vi "PosStrikerAnguloGol.vi"(9 "atacando contra":bool, 10 "IA State":T1={"our_robots"=[], "enemy_robots"=[], "balls"=[], "geometry"={"line_width"=0, "field_length"=0, "field_width"=0, "boundary_width"=0, "referee_width"=0, "goal_width"=0, "goal_depth"=0, "goal_wall_width"=0, "center_circle_radius"=0, "defense_radius"=0, "defense_stretch"=0, "free_kick_from_defense_dist"=0, "penalty_spot_from_field_line_dist"=0, "penalty_line_from_spot_dist"=0}, "IA Judge"={"stage"="", "command"="", "our_goalie_id"=0.0, "enemy_goalie_id"=0.0, "command enum"=enum."Halt", "Time"=enum."Azul"}, "Received Timestamp"=timestamp(0 s since 1904-01-01), "Events"={"Touch"=FALSE, "Ball out"=FALSE, "id touch"=0.0, "Ball out of \nVision"=FALSE, "Ball inside \nGoalie area"=FALSE, "Robot not responding"=FALSE, "Robots responding status"=[1.0, 1.0, 1.0, 1.0, 1.0, 1.0], "Enemy Ball \nPossession"=FALSE, "Pass State"=FALSE, "id end of pass"=0.0, "Kick"=FALSE, "Id ini Possession"=0.0, "Ball Possesion"=FALSE, "Id Possesion"=0.0}}) -> (2 "theta final":dbl)   [LabVIEW 2017]
uses:
  Core/AI Input.ctl
  Core/AI Robot.ctl
  Intel/Functions Enum.ctl
  Intel/AttackerStates.ctl
  Core/AI Ball.ctl
  Core/Field Size.ctl
  Core/AI Judge.ctl
  Intel/Command Enum.ctl
  Events/Events.ctl
panel:
  in  "XdoAttacker":dbl
  in  "YdoAttacker":dbl
  in  "Array":dbl[](array[numeric])=[0.0, 0.0, 0.0, 0.0, 0.0, 0.0]
  in  "Contador 2":dbl
  in  "fim do intervalo":dbl=-1.57
  in  "inicio do intervalo":dbl=-1.57
  in  "tamanho do intervalo":dbl
  in  "valor de theta":dbl
  in  "RobôsParaAnalisar":dbl[][](array[numeric])=[[99999.0, 99999.0], [99999.0, 99999.0], [99999.0, 99999.0], [99999.0, 99999.0], [99999.0, 99999.0], [99999.0, 99999.0], [99999.0, 99999.0]]
  in  "Contador":dbl
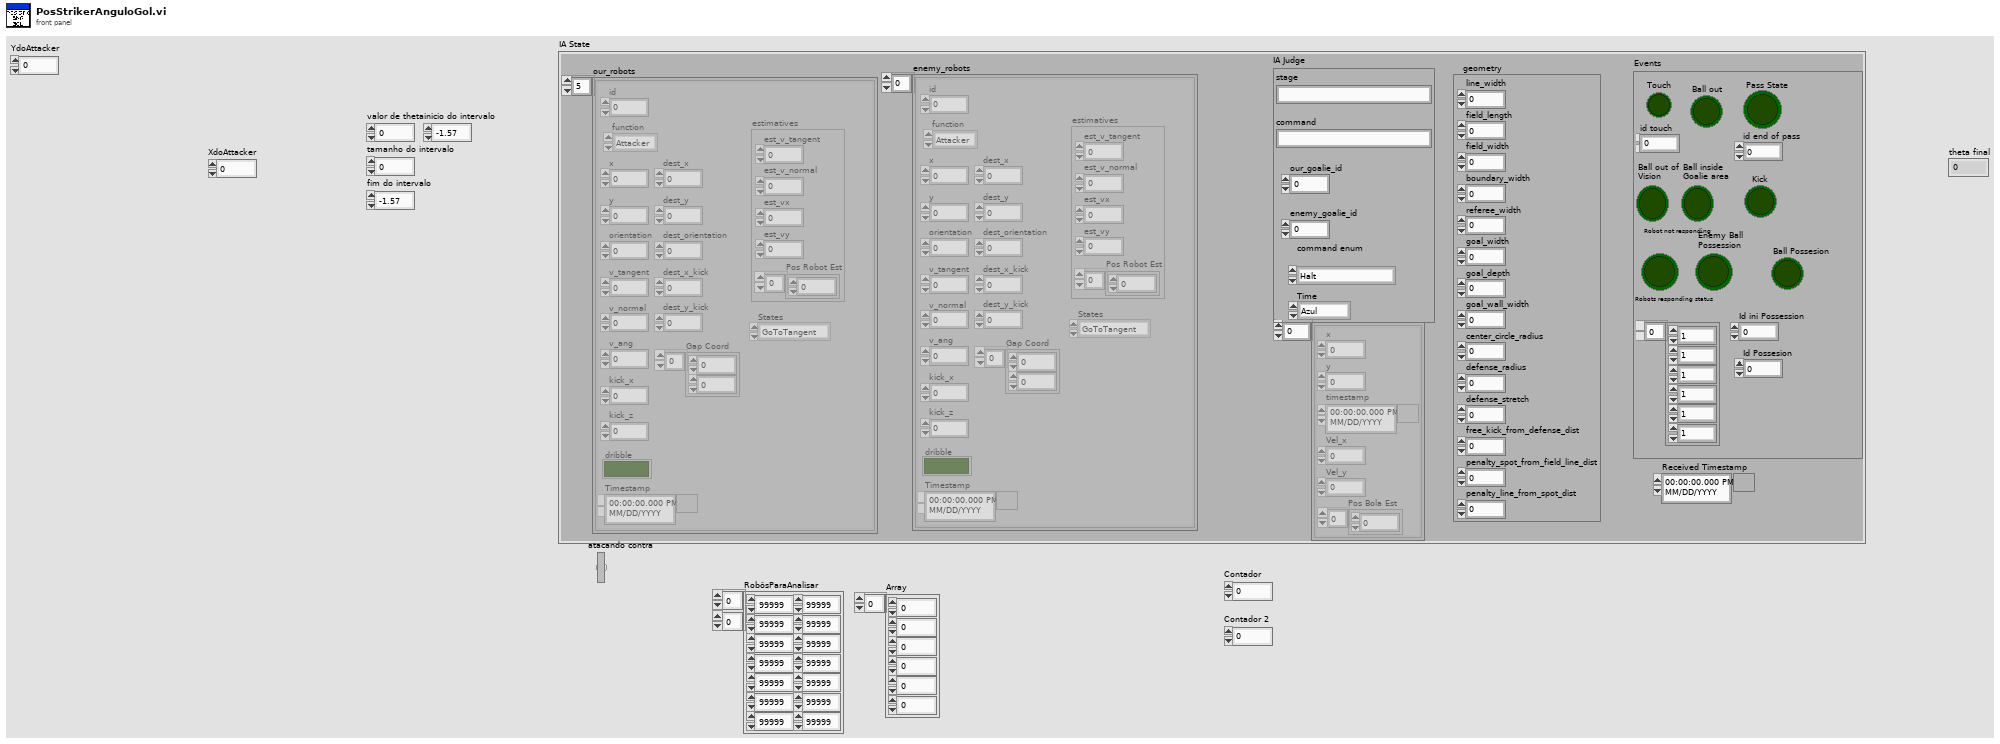
[diagram p1: front panel]
types:
  T1 = typedef "AI Input.ctl" = cluster{"our_robots":T2[], "enemy_robots":T2[], "balls":T5[], "geometry":T6, "IA Judge":T7, "Received Timestamp":timestamp, "Events":T9}
  T2 = typedef "AI Robot.ctl" = cluster{"id":u32, "function":T3, "x":dbl, "y":dbl, "orientation":dbl, "v_tangent":dbl, "v_normal":dbl, "v_ang":dbl, "kick_x":dbl, "kick_z":dbl, "dribble":bool, "Timestamp":timestamp, "dest_x":dbl, "dest_y":dbl, "dest_orientation":dbl, "estimatives":cluster{"est_v_tangent":dbl, "est_v_normal":dbl, "est_vx":dbl, "est_vy":dbl, "Pos Robot Est":dbl[]}, "dest_x_kick":dbl, "dest_y_kick":dbl, "Gap Coord":dbl[], "States":T4}
  T3 = typedef "Functions Enum.ctl" = enum16{"Attacker", "Goalie", "Defender", "Striker", "Goto 0", "Dummy", "Kicker", "ZigZag"}
  T4 = typedef "AttackerStates.ctl" = enum16{"Pass", "GoToTangent", "BallGetting", "GoToKick", ""}
  T5 = typedef "AI Ball.ctl" = cluster{"x":dbl, "y":dbl, "timestamp":timestamp, "Vel_x":dbl, "Vel_y":dbl, "Pos Bola Est":dbl[]}
  T6 = typedef "Field Size.ctl" = cluster{"line_width":u32, "field_length":u32, "field_width":u32, "boundary_width":u32, "referee_width":u32, "goal_width":u32, "goal_depth":u32, "goal_wall_width":u32, "center_circle_radius":u32, "defense_radius":u32, "defense_stretch":u32, "free_kick_from_defense_dist":u32, "penalty_spot_from_field_line_dist":u32, "penalty_line_from_spot_dist":u32}
  T7 = typedef "AI Judge.ctl" = cluster{"stage":string, "command":string, "our_goalie_id":dbl, "enemy_goalie_id":dbl, "command enum":T8, "Time":enum16{"Azul", "Amarelo"}}
  T8 = typedef "Command Enum.ctl" = enum16{"Halt", "Stop", "Force Start", "PKA Normal Start", "Prepare Kickoff Ally", "PKE Normal Start", "Prepare Kickoff Enemy", "Prepare Penalty Ally", "PPA Normal Start", "Prepare Penalty Enemy", "PPE Normal Start", "Direct Free Enemy", "Direct Free Ally", "Indirect Free Enemy", "Indirect Free Ally", "Timeout Enemy", "Timeout Ally", "Goal Enemy", "Goal Ally", "Ball Placement Enemy", "Ball Placement Ally", "Normal Half Time", "Extra Time Break", "Extra Half Time", "None", "Post Game"}
  T9 = typedef "Events.ctl" = cluster{"Touch":bool, "Ball out":bool, "id touch":dbl, "Ball out of \nVision":bool, "Ball inside \nGoalie area":bool, "Robot not responding":bool, "Robots responding status":dbl[], "Enemy Ball \nPossession":bool, "Pass State":bool, "id end of pass":dbl, "Kick":bool, "Id ini Possession":dbl, "Ball Possesion":bool, "Id Possesion":dbl}
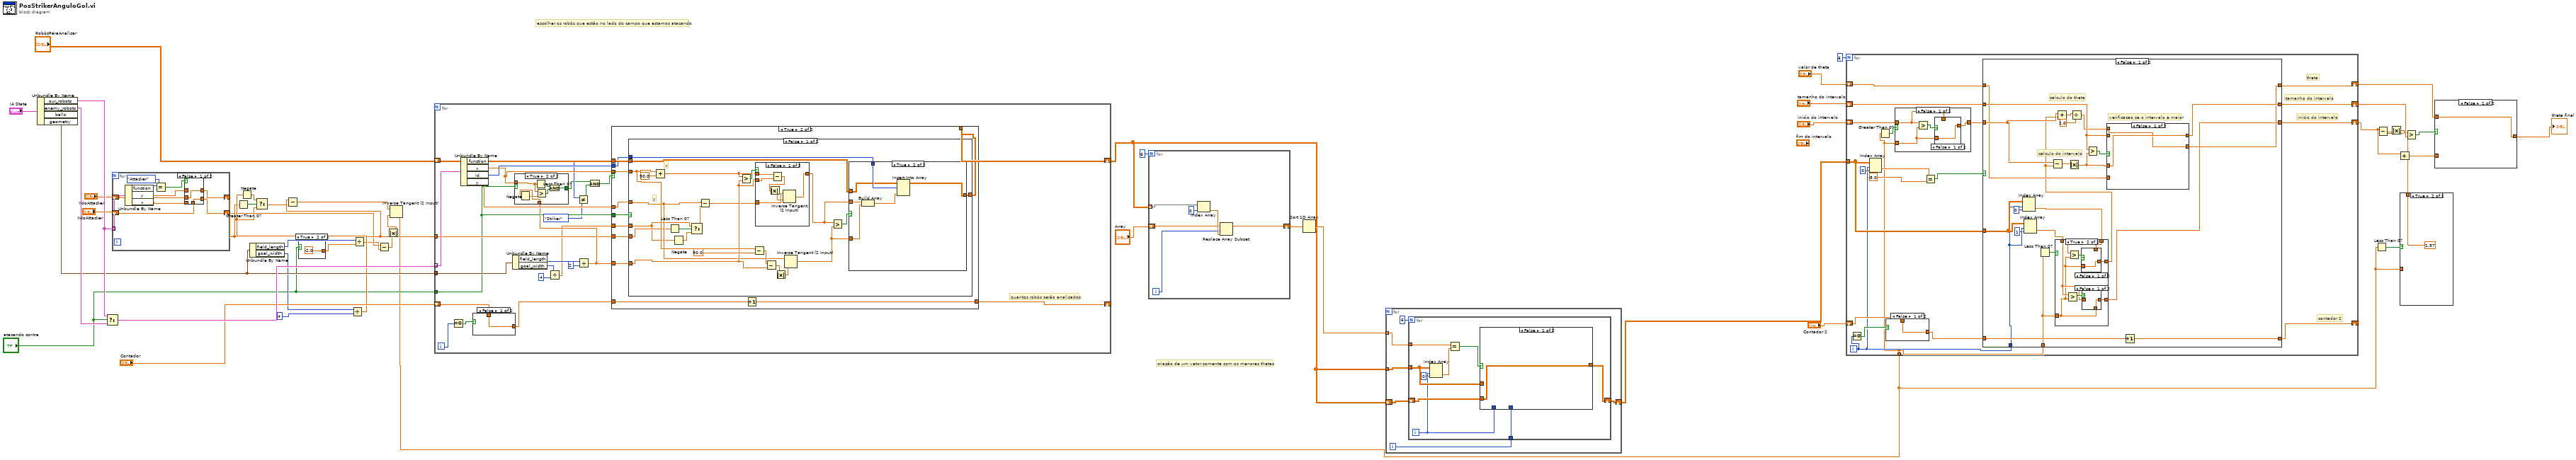
[diagram p0: block diagram]
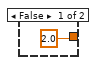
[diagram p3: hidden frame]
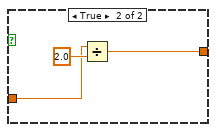
[diagram p5: hidden frame]
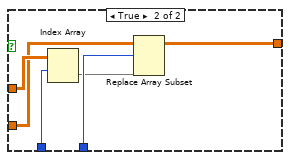
[diagram p6: hidden frame]
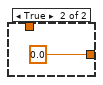
[diagram p9: hidden frame]
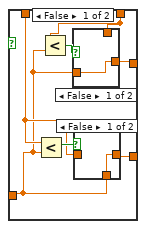
[diagram p10: hidden frame]
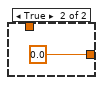
[diagram p17: hidden frame]
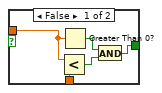
[diagram p18: hidden frame]
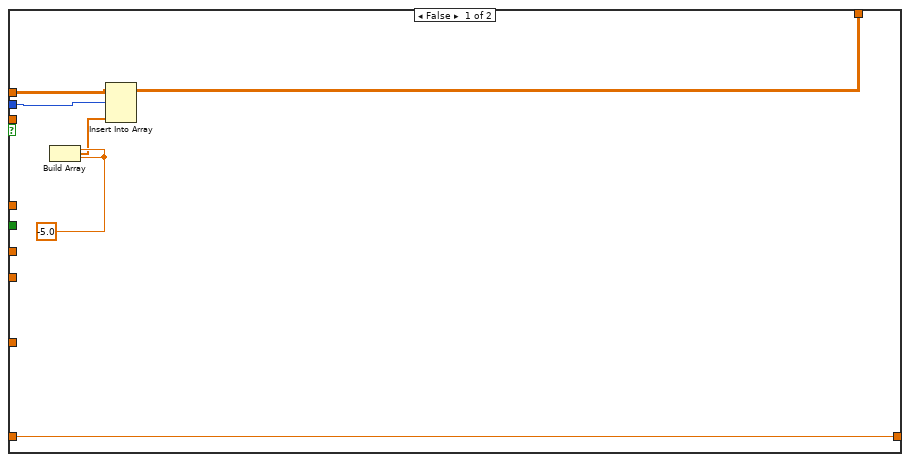
[diagram p19: hidden frame]
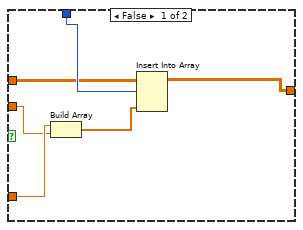
[diagram p20: hidden frame]
diagram:
  # "criação de um vetor somente com os menores thetas"
  # "escolher os robôs que estão no lado do campo que estamos atacando"
  n1 = Unbundle By Name("IA State") -> ("our_robots"=w21:T2[], "enemy_robots"=w45:T2[], "geometry"=w18:T6)  [unwired: 1 out]
  n2 = Select(t=w21, s="atacando contra", f=w45) -> (s? t:f=w44:T2[])
  n3 = for {
    tunnel: w21 -> [w56] mode=indexing
    shift-right: [w51] -> w11
    shift-left: "YdoAttacker" -> [w50]
    shift-right: [w48] -> w8
    shift-left: "XdoAttacker" -> [w47]
    n4 = Unbundle By Name(w56) -> ("function"=w55:T3, "y"=w52:dbl, "x"=w49:dbl)
    n5 = Equal?(x=w55, y=Functions_Enum."Attacker") -> (x = y?=w53:bool)
    n6 = case shown="False" w53 {
      tunnel: w52 -> [_ w60]
      tunnel: [w58 w60] -> w51
      tunnel: w50 -> [w58 _]
      tunnel: w49 -> [_ w59]
      tunnel: [w57 w59] -> w48
      tunnel: w47 -> [w57 _]
      frame False {
      }
      frame True {
      }
    }
  }
  n7 = Greater Than 0?(x=w11) -> (x > 0?=w14:bool)
  n8 = Unbundle By Name(w18) -> ("field_length"=w15:u32, "goal_width"=w17:u32)
  n9 = case shown="True" "atacando contra" {
    tunnel: [2.0 ("y") -2.0 ("y")] -> w6
    frame False {
    }
    frame True {
    }
  }
  n10 = Divide(x=w17, y=u32 4) -> (x/y=w12:dbl)
  n11 = Negate(x=w12) -> (-x=w13:dbl)
  n12 = Select(t=w13, s=w14, f=w12) -> (s? t:f=w10:dbl)
  n13 = Subtract(x=w11, y=w10) -> (x-y=w7:dbl)
  n14 = Divide(x=w15, y=w6) -> (x/y=w9:dbl)
  n15 = Subtract(x=w8, y=w9) -> (x-y=w2:dbl)
  n16 = Absolute Value(x=w2) -> (abs(x)=w1:dbl)
  n17 = Inverse Tangent (2 Input)(1:w1, 2:w7) -> (0:w3:dbl)
  n18 = for {
    tunnel: w44 -> [w87] mode=indexing
    tunnel: "atacando contra" -> [w69]
    shift-right: [w77] -> w32
    shift-left: "RobôsParaAnalisar" -> [w86]
    shift-right: [w78] -> _
    shift-left: "Contador" -> [w80]
    tunnel: w18 -> [w70]
    tunnel: w11 -> [w74]
    i -> [w81]
    # "quantos robôs serão analisados"
    n19 = Equal To 0?(x=w81) -> (x = 0?=w82:bool)
    n20 = Unbundle By Name(w87) -> ("function"=w67:T3, "x"=w84:dbl, "id"=w85:u32, "y"=w83:dbl)
    n21 = case shown="False" w82 {
      tunnel: w80 -> [w88 _]
      tunnel: [w88 0.0] -> w79
      frame False {
      }
      frame True {
      }
    }
    n22 = Unbundle By Name(w70) -> ("field_length"=w76:u32, "goal_width"=w73:u32)
    n23 = Divide(x=w73, y=u32 4) -> (x/y=w71:dbl)
    n24 = Not Equal?(x=w67, y=Functions_Enum."Striker") -> (x != y?=w64:bool)
    n25 = Divide(x=w76, y=u32 2) -> (x/y=w75:dbl)
    n26 = case shown="True" w69 {
      tunnel: w84 -> [w94 w95]
      tunnel: [w90 w100] -> w63
      tunnel: w75 -> [w93 w96]
      frame False {
        n27 = Less?(x=w94, y=w93) -> (x < y?=w91:bool)
        n28 = Greater Than 0?(x=w94) -> (x > 0?=w92:bool)
        n29 = And(x=w92, y=w91) -> (x .and. y?=w90:bool)
      }
      frame True {
        n30 = Negate(x=w96) -> (-x=w97:dbl)
        n31 = Less Than 0?(x=w95) -> (x < 0?=w99:bool)
        n32 = Greater?(x=w95, y=w97) -> (0:w98:bool)
        n33 = And(x=w99, y=w98) -> (x .and. y?=w100:bool)
      }
    }
    n34 = And(x=w63, y=w64) -> (x .and. y?=w65:bool)
    n35 = case shown="True" w65 {
      tunnel: w86 -> [w105 w112]
      tunnel: w85 -> [w104 w110]
      tunnel: w84 -> [_ w114]
      tunnel: w83 -> [_ w111]
      tunnel: w79 -> [w106 w116]
      tunnel: [w106 w117] -> w78
      tunnel: [w101 w109] -> w77
      tunnel: w69 -> [_ w115]
      tunnel: w75 -> [_ w113]
      tunnel: w74 -> [_ w108]
      tunnel: w71 -> [_ w107]
      frame False {
        w103 = -5.0 ("element")
        n36 = Build Array(w103, w103) -> (w102:dbl[])
        n37 = Insert Into Array(array=w105, index (row)=w104, new element=w102) -> (w101:dbl[][])  [unwired: 1 in]
      }
      frame True {
        n38 = case shown="False" w115 {
          tunnel: w114 -> [w129 w177]
          tunnel: w113 -> [w128 w180]
          tunnel: w112 -> [w130 w172]
          tunnel: w111 -> [w121 w161]
          tunnel: w110 -> [w131 w171]
          tunnel: [w127 w168] -> w109
          tunnel: w108 -> [w120 w165]
          tunnel: w107 -> [w119 w162]
          frame False {
            # "y"
            # "x"
            n39 = Add(x=w129, y=90.0) -> (x+y=w137:dbl)
            n40 = Less Than 0?(x=w120) -> (x < 0?=w124:bool)
            n41 = Negate(x=w119) -> (-x=w123:dbl)
            n42 = Select(t=w119, s=w124, f=w123) -> (s? t:f=w122:dbl)
            n43 = Subtract(x=w121, y=w122) -> (x-y=w118:dbl)
            n44 = Greater?(x=w137, y=w128) -> (0:w138:bool)
            n45 = Subtract(x=w129, y=90.0) -> (x-y=w135:dbl)
            n46 = case shown="False" w138 {
              tunnel: w137 -> [w157 _]
              tunnel: [w154 1.57] -> w133
              tunnel: w128 -> [w156 _]
              tunnel: w118 -> [w155 _]
              frame False {
                n47 = Subtract(x=w157, y=w156) -> (x-y=w153:dbl)
                n48 = Absolute Value(x=w153) -> (abs(x)=w152:dbl)
                n49 = Inverse Tangent (2 Input)(1:w152, 2:w155) -> (0:w154:dbl)
              }
              frame True {
              }
            }
            n50 = Subtract(x=w135, y=w128) -> (x-y=w125:dbl)
            n51 = Absolute Value(x=w125) -> (abs(x)=w126:dbl)
            n52 = Inverse Tangent (2 Input)(1:w126, 2:w121) -> (0:w132:dbl)
            n53 = Greater?(x=w133, y=w132) -> (0:w134:bool)
            n54 = case shown="True" w134 {
              tunnel: w130 -> [w142 w148]
              tunnel: w131 -> [w144 w151]
              tunnel: w133 -> [w141 w149]
              tunnel: w132 -> [w143 w147]
              tunnel: [w140 w146] -> w127
              frame False {
                n55 = Build Array(w143, w141) -> (w145:dbl[])
                n56 = Insert Into Array(array=w142, index (row)=w144, new element=w145) -> (w140:dbl[][])  [unwired: 1 in]
              }
              frame True {
                n57 = Build Array(w149, w147) -> (w150:dbl[])
                n58 = Insert Into Array(array=w148, index (row)=w151, new element=w150) -> (w146:dbl[][])  [unwired: 1 in]
              }
            }
          }
          frame True {
            # "y"
            # "x"
            n59 = Negate(x=w180) -> (-x=w174:dbl)
            n60 = Subtract(x=w177, y=90.0) -> (x-y=w178:dbl)
            n61 = Greater Than 0?(x=w165) -> (x > 0?=w164:bool)
            n62 = Negate(x=w162) -> (-x=w163:dbl)
            n63 = Select(t=w162, s=w164, f=w163) -> (s? t:f=w160:dbl)
            n64 = Subtract(x=w161, y=w160) -> (x-y=w159:dbl)
            n65 = Less?(x=w178, y=w174) -> (x < y?=w179:bool)
            n66 = Add(x=w177, y=90.0) -> (x+y=w175:dbl)
            n67 = case shown="False" w179 {
              tunnel: w178 -> [w199 _]
              tunnel: [w196 1.57] -> w170
              tunnel: w174 -> [w198 _]
              tunnel: w159 -> [w197 _]
              frame False {
                n68 = Subtract(x=w199, y=w198) -> (x-y=w194:dbl)
                n69 = Absolute Value(x=w194) -> (abs(x)=w195:dbl)
                n70 = Inverse Tangent (2 Input)(1:w195, 2:w197) -> (0:w196:dbl)
              }
              frame True {
              }
            }
            n71 = Subtract(x=w175, y=w174) -> (x-y=w166:dbl)
            n72 = Absolute Value(x=w166) -> (abs(x)=w167:dbl)
            n73 = Inverse Tangent (2 Input)(1:w167, 2:w161) -> (0:w169:dbl)
            n74 = Greater?(x=w170, y=w169) -> (0:w173:bool)
            n75 = case shown="True" w173 {
              tunnel: w172 -> [w184 w190]
              tunnel: w171 -> [w186 w193]
              tunnel: w170 -> [w183 w191]
              tunnel: w169 -> [w185 w189]
              tunnel: [w182 w188] -> w168
              frame False {
                n76 = Build Array(w185, w183) -> (w187:dbl[])
                n77 = Insert Into Array(array=w184, index (row)=w186, new element=w187) -> (w182:dbl[][])  [unwired: 1 in]
              }
              frame True {
                n78 = Build Array(w191, w189) -> (w192:dbl[])
                n79 = Insert Into Array(array=w190, index (row)=w193, new element=w192) -> (w188:dbl[][])  [unwired: 1 in]
              }
            }
          }
        }
        n80 = Increment(x=w116) -> (x+1=w117:dbl)
      }
    }
  }
  n81 = for {
    N: 6 -> [_]
    tunnel: w32 -> [w206] mode=indexing
    shift-right: [w201] -> w34
    shift-left: "Array" -> [w202]
    i -> [w203]
    n82 = Index Array(array=w206, index=0) -> (element=w204:dbl)
    n83 = Replace Array Subset(array=w202, new element=w204, index=w203) -> (w201:dbl[])
  }
  n84 = Sort 1D Array(array=w34) -> (sorted array=w33:dbl[])
  n85 = for {
    tunnel: w33 -> [w209] mode=indexing
    tunnel: w32 -> [w211]
    shift-right: [w207] -> w31
    shift-left: w32 -> [w210]
    i -> [w208]
    n86 = for {
      N: 6 -> [_]
      tunnel: w211 -> [w217]
      shift-right: [w213] -> w207
      shift-left: w210 -> [w216]
      tunnel: w209 -> [w219]
      tunnel: w208 -> [w214]
      i -> [w215]
      n87 = Index Array(array=w217, index (row)=w215, index (col)=0 ("disabled index (col)")) -> (element=w220:dbl)
      n88 = Equal?(x=w219, y=w220) -> (x = y?=w218:bool)
      n89 = case shown="False" w218 {
        tunnel: w217 -> [_ w228]
        tunnel: w216 -> [w222 w224]
        tunnel: w215 -> [_ w227]
        tunnel: w214 -> [_ w226]
        tunnel: [w222 w223] -> w213
        frame False {
        }
        frame True {
          n90 = Index Array(array=w228, index (row)=w227) -> (element=w225:dbl[])  [unwired: 1 in]
          n91 = Replace Array Subset(array=w224, new element=w225, index (row)=w226) -> (w223:dbl[][])  [unwired: 1 in]
        }
      }
    }
  }
  n92 = for {
    N: 6 -> [_]
    tunnel: w31 -> [w236]
    shift-right: [w244] -> w27
    shift-left: "valor de theta" -> [w245]
    shift-right: [w242] -> w30
    shift-left: "tamanho do intervalo" -> [w243]
    shift-right: [w241] -> w24
    shift-left: "inicio do intervalo" -> [w230]
    shift-right: [w237] -> _
    shift-left: "Contador 2" -> [w239]
    tunnel: w3 -> [w229]
    i -> [w235]
    # "contador 2"
    # "inicio do intervalo"
    # "tamanho do intervalo"
    # "theta"
    n93 = Equal To 0?(x=w235) -> (x = 0?=w240:bool)
    n94 = Index Array(array=w236, index (row)=w235, index (col)=0 ("disabled index (col)")) -> (element=w234:dbl)
    n95 = Greater Than 0?(x=w229) -> (x > 0?=w232:bool)
    n96 = case shown="False" w240 {
      tunnel: w239 -> [w255 _]
      tunnel: [w255 0.0] -> w238
      frame False {
      }
      frame True {
      }
    }
    n97 = case shown="False" w232 {
      tunnel: [w250 w254] -> w231
      tunnel: w230 -> [w249 w254]
      tunnel: w229 -> [w248 _]
      frame False {
        n98 = Greater?(x=w249, y=w248) -> (0:w251:bool)
        n99 = case shown="False" w251 {
          tunnel: [w252 w253] -> w250
          tunnel: w249 -> [_ w253]
          tunnel: w248 -> [w252 _]
          frame False {
          }
          frame True {
          }
        }
      }
      frame True {
      }
    }
    n100 = Equal?(x=w234, y=-5.0) -> (x = y?=w233:bool)
    n101 = case shown="False" w233 {
      tunnel: w245 -> [w263 w309]
      tunnel: [w264 w309] -> w244
      tunnel: w243 -> [w268 w308]
      tunnel: [w267 w308] -> w242
      tunnel: w231 -> [w279 w307]
      tunnel: [w257 w307] -> w241
      tunnel: w238 -> [w277 w306]
      tunnel: [w278 w306] -> w237
      tunnel: w236 -> [w276 _]
      tunnel: w235 -> [w275 _]
      tunnel: w229 -> [w261 _]
      frame False {
        # "calculo do theta"
        # "calculo do intervalo"
        # "verificacao se o intervalo é maior"
        n102 = Index Array(array=w276, index (row)=w275, index (col)=0 ("disabled index (col)")) -> (element=w260:dbl)
        n103 = Index Array(array=w276, index (row)=w275, index (col)=1 ("disabled index (col)")) -> (element=w258:dbl)
        n104 = Less Than 0?(x=w261) -> (x < 0?=w262:bool)
        n105 = case shown="True" w262 {
          tunnel: w258 -> [w284 w293]
          tunnel: w260 -> [w280 w295]
          tunnel: w261 -> [w283 w291]
          tunnel: [w282 w296] -> w259
          tunnel: [w281 w292] -> w257
          frame False {
            n106 = Less?(x=w284, y=w283) -> (x < y?=w286:bool)
            n107 = Less?(x=w280, y=w283) -> (x < y?=w285:bool)
            n108 = case shown="False" w285 {
              tunnel: [w289 w290] -> w282
              tunnel: w280 -> [_ w290]
              tunnel: w283 -> [w289 _]
              frame False {
              }
              frame True {
              }
            }
            n109 = case shown="False" w286 {
              tunnel: w284 -> [_ w288]
              tunnel: [w287 w288] -> w281
              tunnel: w283 -> [w287 _]
              frame False {
              }
              frame True {
              }
            }
          }
          frame True {
            n110 = Greater?(x=w293, y=w291) -> (0:w294:bool)
            n111 = Greater?(x=w295, y=w291) -> (0:w297:bool)
            n112 = case shown="False" w297 {
              tunnel: [w300 w301] -> w296
              tunnel: w295 -> [_ w301]
              tunnel: w291 -> [w300 _]
              frame False {
              }
              frame True {
              }
            }
            n113 = case shown="False" w294 {
              tunnel: w293 -> [_ w299]
              tunnel: [w298 w299] -> w292
              tunnel: w291 -> [w298 _]
              frame False {
              }
              frame True {
              }
            }
          }
        }
        n114 = Subtract(x=w279, y=w259) -> (x-y=w272:dbl)
        n115 = Add(x=w279, y=w259) -> (x+y=w271:dbl)
        n116 = Absolute Value(x=w272) -> (abs(x)=w266:dbl)
        n117 = Divide(x=w271, y=2.0) -> (x/y=w265:dbl)
        n118 = Greater?(x=w268, y=w266) -> (0:w269:bool)
        n119 = case shown="False" w269 {
          tunnel: w268 -> [_ w305]
          tunnel: [w303 w305] -> w267
          tunnel: w266 -> [w303 _]
          tunnel: w263 -> [_ w304]
          tunnel: w265 -> [w302 _]
          tunnel: [w302 w304] -> w264
          frame False {
          }
          frame True {
          }
        }
        n120 = Increment(x=w277) -> (x+1=w278:dbl)
      }
      frame True {
      }
    }
  }
  n121 = Less Than 0?(x=w3) -> (x < 0?=w4:bool)
  n122 = case shown="True" w4 {
    tunnel: [w310 1.57 ("y")] -> w23
    tunnel: w3 -> [w310 _]
    frame False {
    }
    frame True {
    }
  }
  n123 = Subtract(x=w24, y=w23) -> (x-y=w26:dbl)
  n124 = Absolute Value(x=w26) -> (abs(x)=w25:dbl)
  n125 = Add(x=w24, y=w23) -> (x+y=w22:dbl)
  n126 = Greater?(x=w25, y=w30) -> (0:w29:bool)
  n127 = case shown="False" w29 {
    tunnel: [w312 w314] -> w28
    tunnel: w27 -> [w312 _]
    tunnel: w22 -> [_ w313]
    frame False {
    }
    frame True {
      n128 = Divide(x=w313, y=2.0) -> (x/y=w314:dbl)
    }
  }
  "theta final" <- w28
